vi "Get All TableVariablet.vi"(8 "error in (no error)":errorcluster, 11 "DataTable":refnum<k7>) -> (0 "error out":errorcluster, 3 "DataTable out":refnum<k7>)   [LabVIEW 2019, in "JMP Automation.lvlib"]
doc: "retreive the name list of the TableVariable from a DataTable. The DataTable will be \"activated\" (put on the front) during the opperation\n\nDataTable: valide DataTable application handle"
uses:
  <instrlib>/LV_JMP_bridge/JMP Automation.lvlib
panel:
  out "Array":string[](array[string])
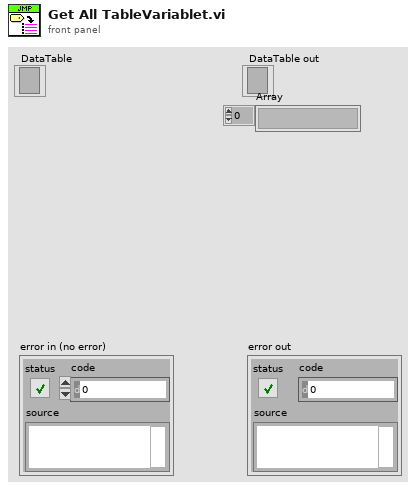
[diagram p1: front panel]
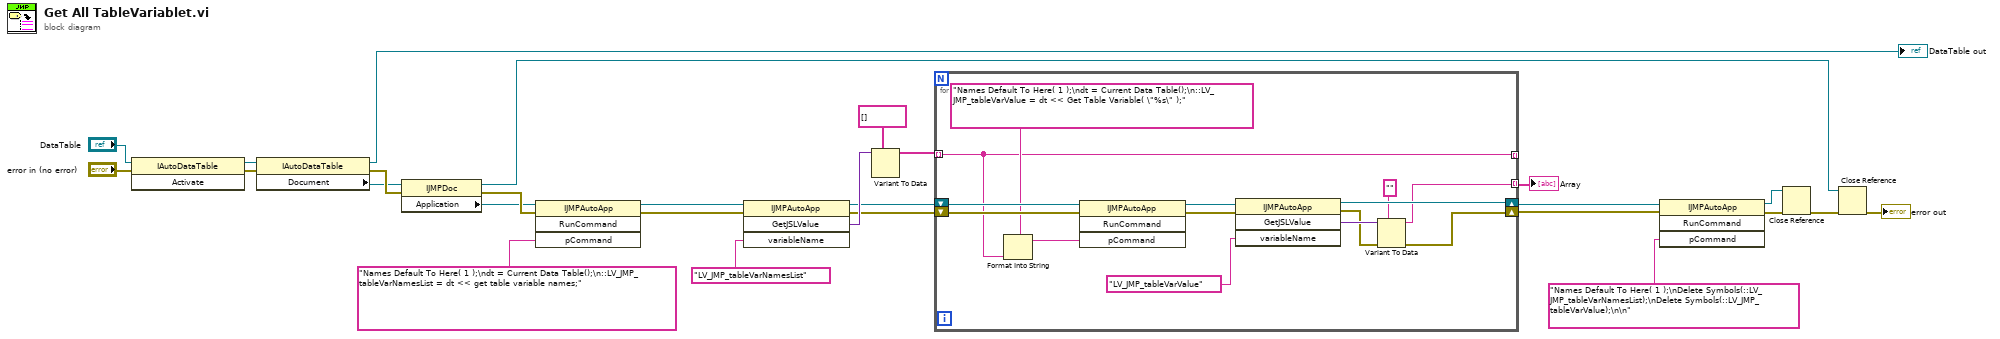
[diagram p0: block diagram]
diagram:
  n1 = invoke class="IAutoDataTable" method="Activate"(reference="DataTable", error in="error in (no error)") -> (reference out=w3:refnum<k7>, error out=w2:errorcluster)  [unwired: 1 in, 1 out]
  n2 = property class="IAutoDataTable"(reference=w3, error in=w2) -> (reference out=→"DataTable out":refnum<k7>, error out=w12:errorcluster, "Document"=w10:refnum<k7>)
  n3 = property class="IJMPDoc"(reference=w10, error in=w12) -> (reference out=w9:refnum<k7>, error out=w13:errorcluster, "Application"=w11:refnum<k7>)
  n4 = invoke class="IJMPAutoApp" method="RunCommand"(reference=w11, error in=w13, "pCommand"="Names Default To Here( 1 );\ndt = Current Data Table();\n::LV_JMP_tableVarNamesList = dt << get table variable names;") -> (reference out=w17:refnum<k7>, error out=w18:errorcluster)  [unwired: 1 in, 2 out]
  n5 = invoke class="IJMPAutoApp" method="GetJSLValue"(reference=w17, error in=w18, "variableName"="LV_JMP_tableVarNamesList") -> (reference out=w19:refnum<k7>, error out=w20:errorcluster, "GetJSLValue"=w21:variant)  [unwired: 1 in, 1 out]
  n6 = Variant To Data(type=string[] [], Variant=w21) -> (data=w22:string[])  [unwired: 1 in, 1 out]
  n7 = for {
    shift-right: [w31] -> w8
    shift-left: w19 -> [w41]
    shift-right: [w32] -> w7
    shift-left: w20 -> [w40]
    tunnel: w22 -> [w28] mode=indexing
    tunnel: [w30] -> w1 mode=indexing
    tunnel: [w28] -> _ mode=indexing
    n8 = Format Into String(initial string="Names Default To Here( 1 );\ndt = Current Data Table();\n::LV_JMP_tableVarValue = dt << Get Table Variable( \"%s\" );", w28) -> (resulting string=w39:string)  [unwired: 2 in, 1 out]
    n9 = invoke class="IJMPAutoApp" method="RunCommand"(reference=w41, error in=w40, "pCommand"=w39) -> (reference out=w37:refnum<k7>, error out=w35:errorcluster)  [unwired: 1 in, 2 out]
    n10 = invoke class="IJMPAutoApp" method="GetJSLValue"(reference=w37, error in=w35, "variableName"="LV_JMP_tableVarValue") -> (reference out=w31:refnum<k7>, error out=w33:errorcluster, "GetJSLValue"=w34:variant)  [unwired: 1 in, 1 out]
    n11 = Variant To Data(error in=w33, type="", Variant=w34) -> (data=w30:string, error out=w32:errorcluster)
  }
  "Array" <- w1
  n12 = invoke class="IJMPAutoApp" method="RunCommand"(reference=w8, error in=w7, "pCommand"="Names Default To Here( 1 );\nDelete Symbols(::LV_JMP_tableVarNamesList);\nDelete Symbols(::LV_JMP_tableVarValue);\n\n") -> (reference out=w6:refnum<k7>, error out=w5:errorcluster)  [unwired: 1 in, 2 out]
  n13 = Close Reference(reference=w6, error in (no error)=w5) -> (error out=w25:errorcluster)
  n14 = Close Reference(reference=w9, error in (no error)=w25) -> (error out=→"error out":errorcluster)
